vi "Prax12.3.1.vi"(10 "Array":dbl[](array[numeric])) -> (2 "transposed array":dbl[][](array[numeric]))   [LabVIEW 2020]
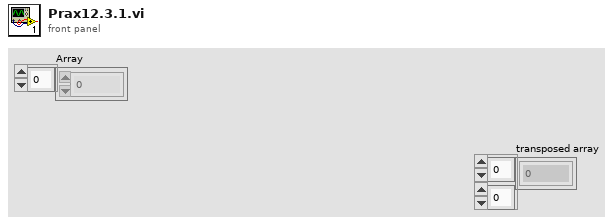
[diagram p1: front panel]
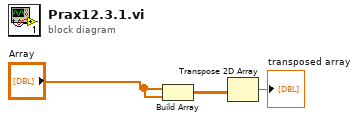
[diagram p0: block diagram]
diagram:
  n1 = Build Array("Array", "Array") -> (w2:dbl[][])
  n2 = Transpose 2D Array(2D array=w2) -> (transposed array=→"transposed array":dbl[][])
